vi "CRYGet Frequency Resolution Param.vi"(8 "Overlap(%)":dbl, 9 "Fs":dbl=44100.0, 10 "Freq Resolution(Hz)":dbl, 11 "Samples":dbl=44100.0) -> (0 "Out Freq Resolution(Hz)":dbl, 1 "Shift Samples":dbl, 2 "No. of FFT":i32, 3 "Record Length(s)":dbl format="%#_6p")   [LabVIEW 2013]
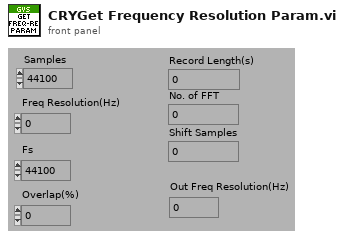
[diagram p1: front panel]
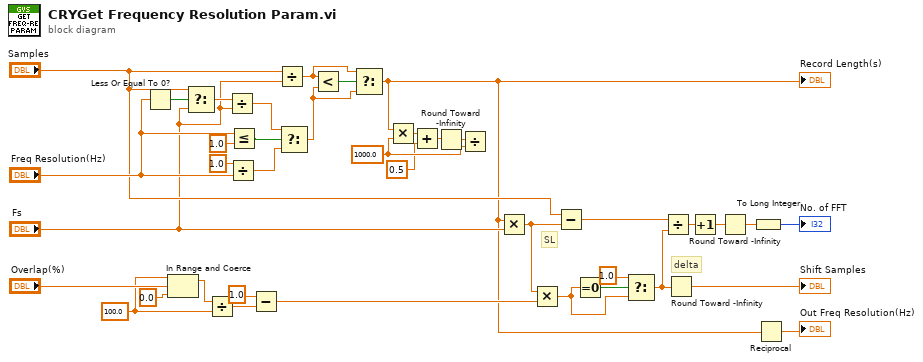
[diagram p0: block diagram]
diagram:
  w7 = 1000.0 ("y")
  w34 = 100.0 ("upper limit")
  # "SL"
  # "delta"
  n1 = Less Or Equal To 0?(x="Freq Resolution(Hz)") -> (x <= 0?=w22:bool)
  n2 = In Range and Coerce(upper limit=w34, x="Overlap(%)", lower limit=0.0) -> (coerced(x)=w35:dbl)  [unwired: 1 out]
  n3 = Select(t="Samples", s=w22, f="Fs") -> (s? t:f=w25:dbl)
  n4 = Divide(x=w35, y=w34) -> (x/y=w20:dbl)
  n5 = Divide(x=w25, y="Fs") -> (x/y=w14:dbl)
  n6 = Divide(x=1.0 ("t"), y="Freq Resolution(Hz)") -> (x/y=w28:dbl)
  n7 = Less Or Equal?(x="Freq Resolution(Hz)", y=1.0) -> (x <= y?=w26:bool)
  n8 = Subtract(x=1.0, y=w20) -> (x-y=w17:dbl)
  n9 = Divide(x="Samples", y="Fs") -> (x/y=w10:dbl)
  n10 = Select(t=w14, s=w26, f=w28) -> (s? t:f=w9:dbl)
  n11 = Less?(x=w10, y=w9) -> (x < y?=w13:bool)
  n12 = Select(t=w10, s=w13, f=w9) -> (s? t:f=w1:dbl)
  "Record Length(s)" <- w1
  n13 = Multiply(x=w1, y=w7) -> (x*y=w5:dbl)
  n14 = Add(x=w5, y=0.5) -> (x+y=w6:dbl)
  n15 = Round Toward -Infinity(1:w6) -> (0:w8:dbl)
  n16 = Divide(x=w8, y=w7) -> ()  [unwired: 1 out]
  n17 = Multiply(x=w1, y="Fs") -> (x*y=w21:dbl)
  n18 = Multiply(x=w21, y=w17) -> (x*y=w16:dbl)
  n19 = Subtract(x="Samples", y=w21) -> (x-y=w15:dbl)
  n20 = Equal To 0?(x=w16) -> (x = 0?=w18:bool)
  n21 = Select(t=1.0, s=w18, f=w16) -> (s? t:f=w3:dbl)
  n22 = Divide(x=w15, y=w3) -> (x/y=w33:dbl)
  n23 = Round Toward -Infinity(1:w3) -> (0:→"Shift Samples":dbl)
  n24 = Increment(x=w33) -> (x+1=w32:dbl)
  n25 = Round Toward -Infinity(1:w32) -> (0:w30:dbl)
  n26 = To Long Integer(number=w30) -> (32bit integer=→"No. of FFT":i32)
  n27 = Reciprocal(x=w1) -> (1/x=→"Out Freq Resolution(Hz)":dbl)
